vi "39-sub.vi"(0 "p":i32) -> (1 "Set":set{i32[]}(c389), 2 "Number of Solutions":i32)   [LabVIEW 2021]
uses:
  2fc8d368-c9e5-4a22-b7d7-51d40e863c15.vi
  <vilib>/Comparison/Less/Less Functor/Less Functor.lvclass
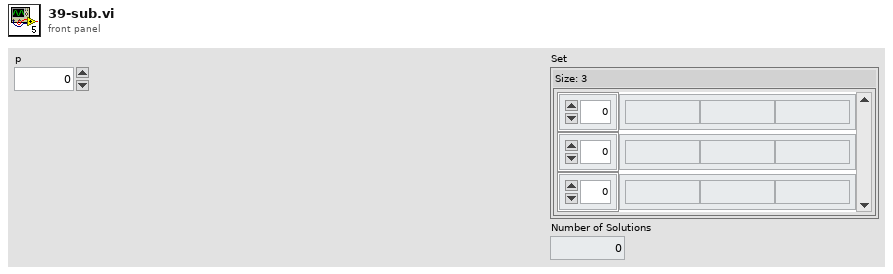
[diagram p1: front panel]
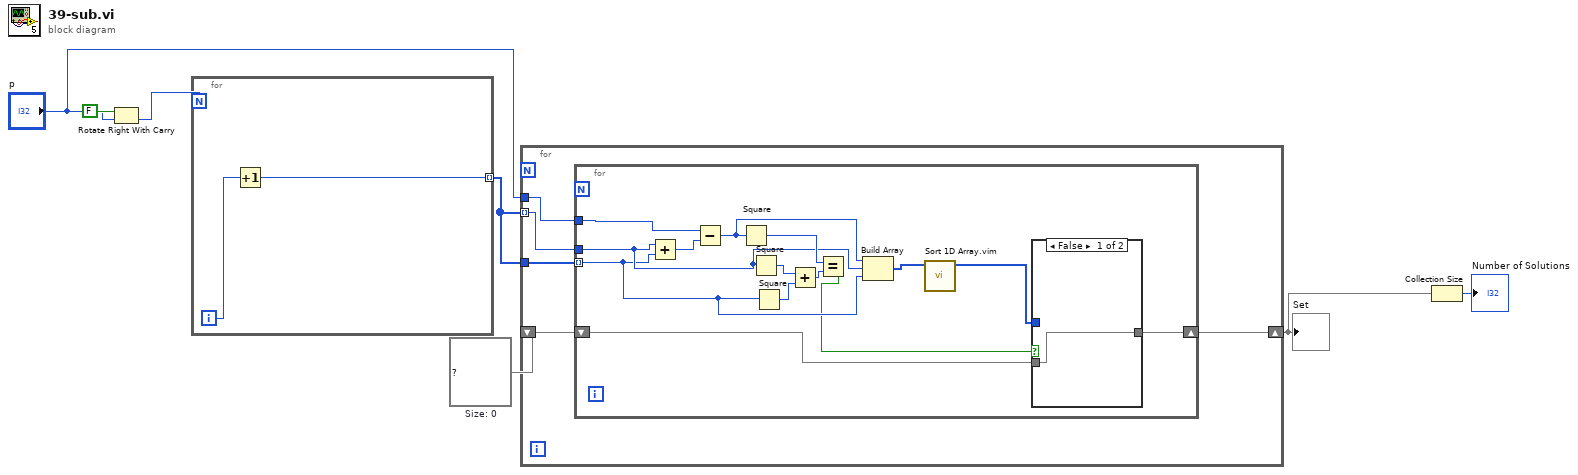
[diagram p0: block diagram]
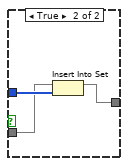
[diagram p2: hidden frame]
diagram:
  w3 = set{i32[]} {}  # Size: 0
  n1 = Rotate Right With Carry(2:"p", 3:FALSE ("carry")) -> (0:w6:i32)  [unwired: 1 out]
  n2 = for {
    N: w6 -> [_]
    tunnel: [w8] -> w5 mode=indexing
    i -> [w9]
    n3 = Increment(x=w9) -> (x+1=w8:i32)
  }
  n4 = for {
    tunnel: w5 -> [w14] mode=indexing
    tunnel: w5 -> [w13]
    tunnel: "p" -> [w12]
    shift-right: [w10] -> w2
    shift-left: w3 -> [w11]
    n5 = for {
      tunnel: w14 -> [w22]
      tunnel: w13 -> [w21] mode=indexing
      tunnel: w12 -> [w27]
      shift-right: [w16] -> w10
      shift-left: w11 -> [w17]
      n6 = Add(x=w22, y=w21) -> (x+y=w28:i32)
      n7 = Subtract(x=w27, y=w28) -> (x-y=w15:i32)
      n8 = Square(x=w15) -> (x^2=w23:i32)
      n9 = Square(x=w22) -> (x^2=w26:i32)
      n10 = Square(x=w21) -> (x^2=w25:i32)
      n11 = Add(x=w26, y=w25) -> (x+y=w24:i32)
      n12 = Equal?(x=w23, y=w24) -> (x = y?=w19:bool)
      n13 = Build Array(w15, w22, w21) -> (w20:i32[])
      n14 = call "Sort 1D Array.vim"("unsorted array"=w20) -> ("sorted array"=w18:i32[])  [unwired: 10 in]
      n15 = case shown="False" w19 {
        tunnel: w18 -> [_ w32]
        tunnel: w17 -> [w29 w31]
        tunnel: [w29 w30] -> w16
        frame False {
        }
        frame True {
          n16 = Insert Into Set(10:w32, 11:w31) -> (3:w30:set{i32[]})  [unwired: 1 out]
        }
      }
    }
  }
  "Set" <- w2
  n17 = Collection Size(1:w2) -> (0:→"Number of Solutions":i32)
